vi "Clear Data Logging Session.vi"(8 "error in (no error)":errorcluster, 10 "Session Name in":string, 11 "Data Logging Manager Ref in":T1) -> (0 "error out":errorcluster, 3 "Data Logging Manager Ref out":T1)   [LabVIEW 2020, in "NI_VS Data Logging API.lvlib"]
uses:
  <vilib>/NI VeriStand/Execution/DataLogging/NI_VS Data Logging API.lvlib
  <vilib>/NI VeriStand/Execution/DataLogging/IDataLogging Ref.ctl
  NationalInstruments.VeriStand.ClientAPI
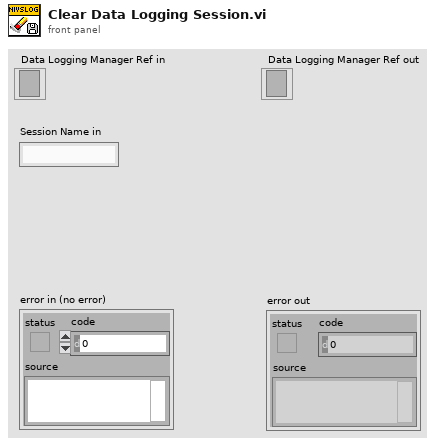
[diagram p1: front panel]
types:
  T1 = typedef "NI_VS Data Logging API.lvlib/IDataLogging Ref.ctl" = refnum<k24>
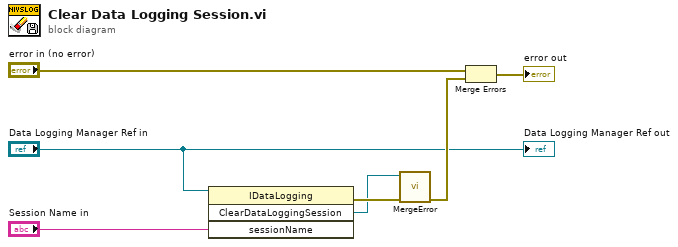
[diagram p0: block diagram]
diagram:
  n1 = invoke class="IDataLogging" method="ClearDataLoggingSession"(reference="Data Logging Manager Ref in", "sessionName"="Session Name in") -> (error out=w5:errorcluster, "ClearDataLoggingSession"=w4:refnum<k24>)  [unwired: 2 in, 2 out]
  n2 = call <vilib>:"MergeError.vi"("error in (no error)"=w5, "Error"=w4) -> ("error out"=w7:errorcluster)  [unwired: 9 out]
  n3 = Merge Errors("error in (no error)", w7) -> (→"error out":errorcluster)
  "Data Logging Manager Ref out" <- "Data Logging Manager Ref in"
